vi "Panel.vi"(11 "DeviceArrayPanel in":refnum<class "DeviceArrayPanel.lvclass">) -> ()   [LabVIEW 2020, in "PicoG-App.lvlib" / "DeviceArrayPanel.lvclass"]
uses:
  DeviceArrayPanel.lvclass
  C:/Program Files (x86)/National Instruments/LabVIEW 2020/vi.lib/IlluminatedG/IG OOPanel/OOPanel/Panel/Panel.lvclass
  <vilib>/IlluminatedG/IG OOPanel/OOPanel/Panel/Basic UI State.ctl
  DeviceArrayPanel.lvclass/DeviceArrayPanel.ctl
  Device/Get ID.vi
  Device/Get Alias.vi
  Device/Get Platform Name.vi
  Device/Get Board.vi
  Device/Get Version String.vi
  <vilib>/IlluminatedG/IG OOPanel/OOPanel/Panel/Panel.lvclass
  <vilib>/IlluminatedG/IG OOPanel/OOPanel/OOPanel.lvlib
  Device/Device.lvclass
panel:
  out "ID":string="E6605838830B8539"
  out "Version String":string="0.0.3"
  out "Board":string="pico"
  out "Platform Name":string="RP2040"
  out "Alias":string="NomadPico"
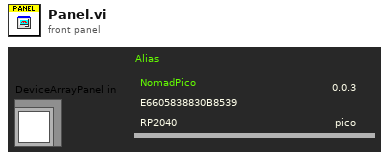
[diagram p1: front panel]
types:
  T1 = typedef "OOPanel.lvlib/Panel.lvclass/Basic UI State.ctl" = enum16{"Init", "Run", "Close"}
  T2 = typedef "PicoG-App.lvlib/DeviceArrayPanel.lvclass/Inbound Events.ctl" = cluster{"Device Set":refnum<user-event>, "Set Highlighted":refnum<user-event>}
  T3 = typedef "OOPanel.lvlib/Panel.lvclass/Panel Events.ctl" = cluster{"Visbility":refnum<user-event>, "Close":refnum<user-event>}
  T4 = typedef "PicoG-App.lvlib/DeviceArrayPanel.lvclass/Ref Data.ctl" = cluster{"Device":refnum<class "Device.lvclass">}
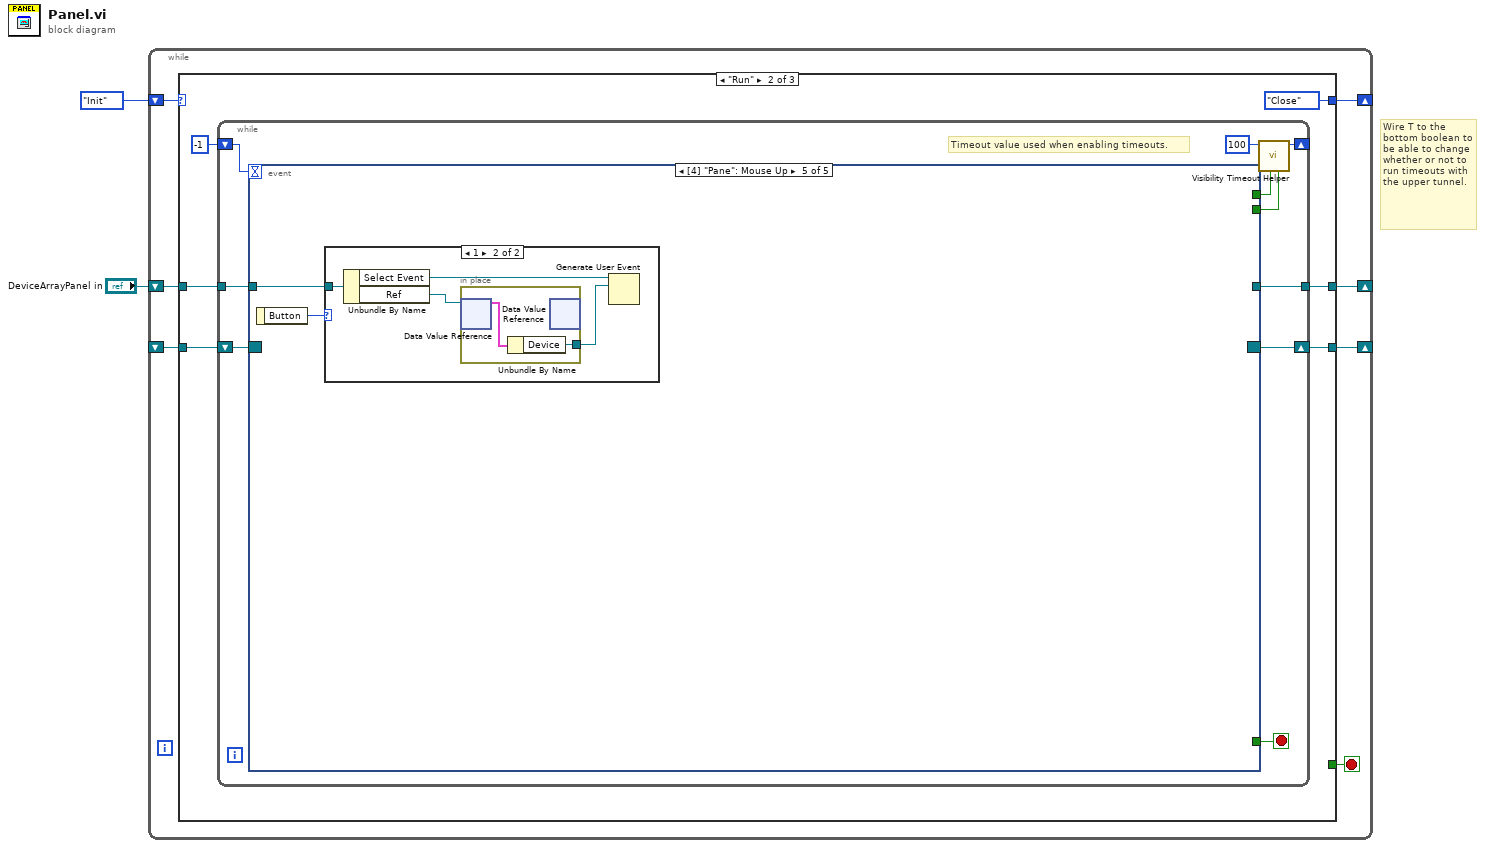
[diagram p0: block diagram]
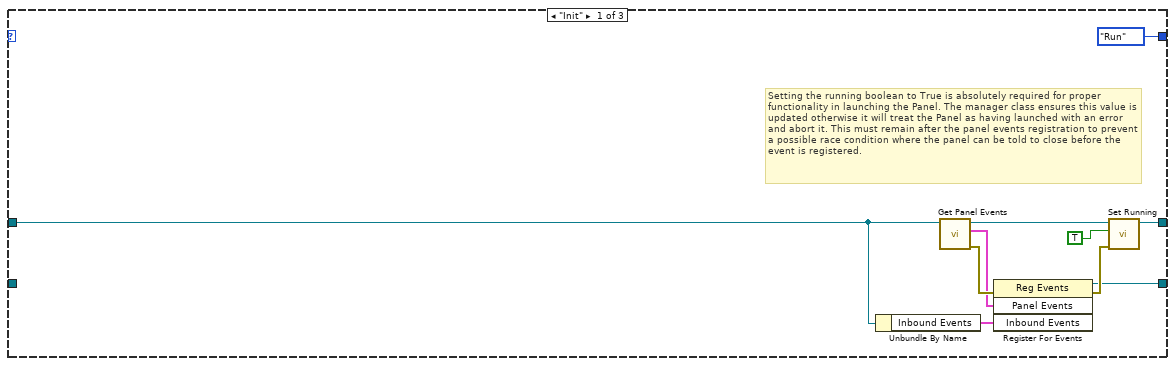
[diagram p2: hidden frame]
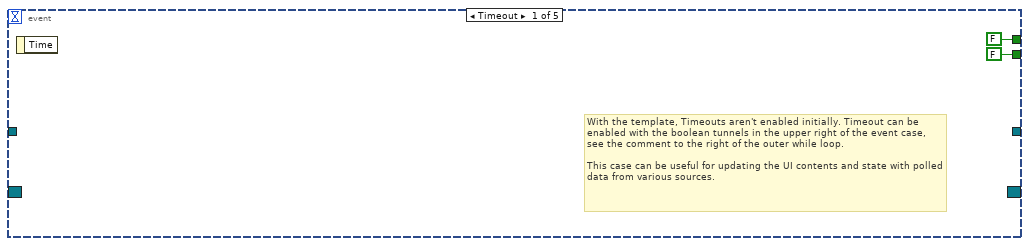
[diagram p3: hidden frame]
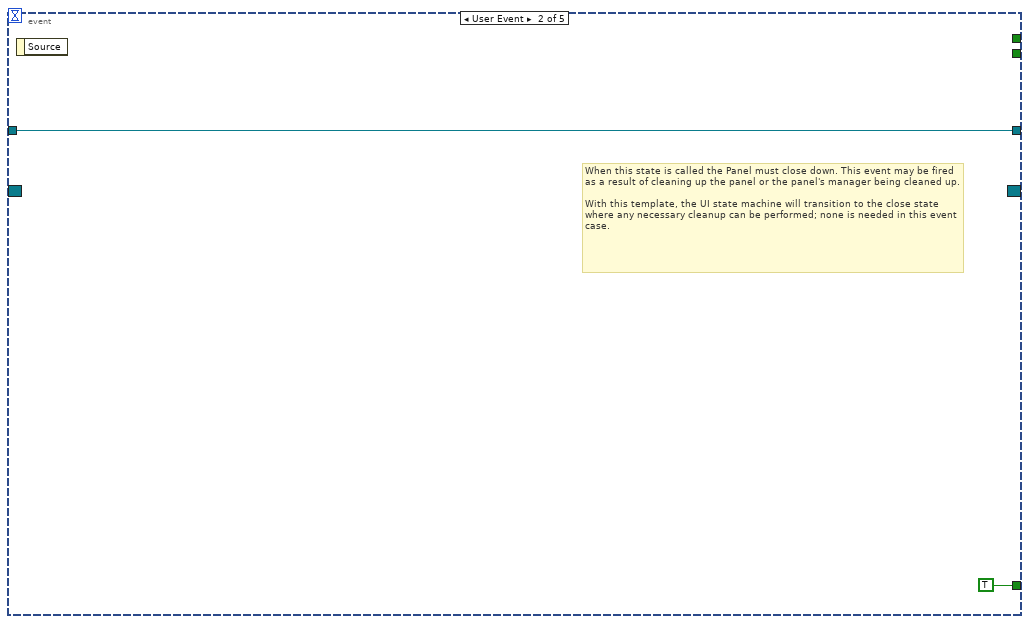
[diagram p4: hidden frame]
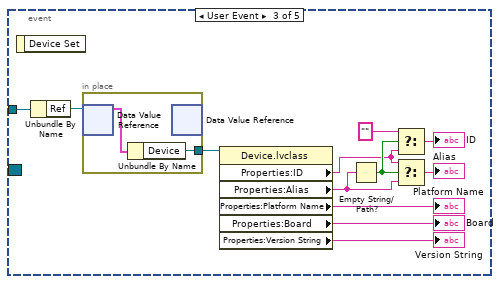
[diagram p5: hidden frame]
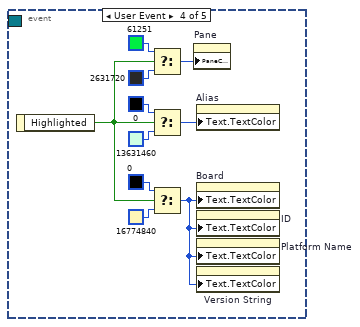
[diagram p6: hidden frame]
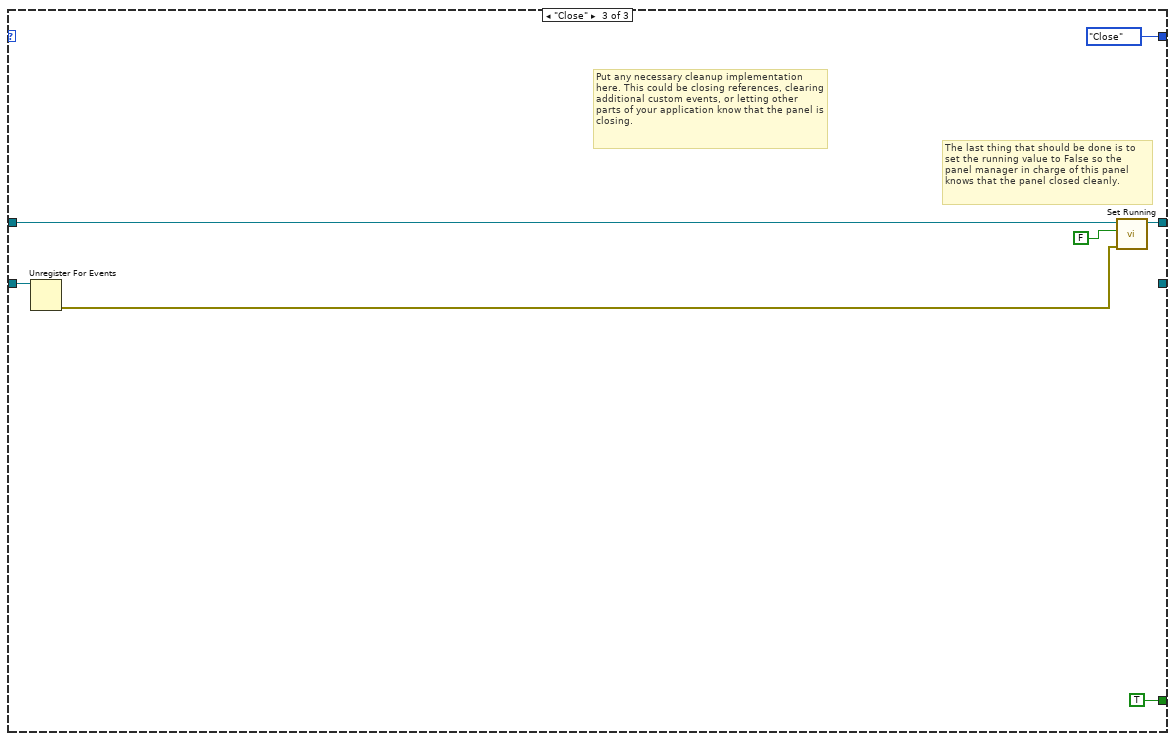
[diagram p8: hidden frame]
diagram:
  # "Wire T to the bottom boolean to be able to change whether or not to run timeouts with the upper tunnel."
  n1 = while {
    shift-right: [w8] -> _
    shift-left: _ -> [w9]
    shift-right: [w6] -> _
    shift-left: Basic_UI_State."Init" ("Basic UI State") -> [w7]
    shift-right: [w4] -> _
    shift-left: "DeviceArrayPanel in" -> [w3]
    stop <- w5 stop-if-true
    n2 = case shown="\"Run\"" w7 {
      tunnel: w9 -> [_ w25 w74]
      tunnel: [w13 w23 _] -> w8
      tunnel: [Basic_UI_State."Run" ("Basic UI State") Basic_UI_State."Close" ("Basic UI State") Basic_UI_State."Close" ("Basic UI State")] -> w6
      tunnel: [_ _ TRUE] -> w5
      tunnel: [w12 w20 w72] -> w4
      tunnel: w3 -> [w11 w21 w73]
      frame "Init" {
        # "Setting the running boolean to True is absolutely required for proper functionality in launching the Panel. The manager class ensures this value is updated otherwise it will treat the Panel as having launched with an error and abort it. This must remain after the panel events registration to prevent a possible race condition where the panel can be told to close before the event is registered."
        n3 = Unbundle By Name(w11) -> ("Inbound Events"=w10:T2)
        n4 = call <vilib>:"Get Panel Events.vi"("Panel in"=w11) -> ("error out"=w19:errorcluster, "Panel Events"=w15:T3, "Panel out"=w16:refnum<class "DeviceArrayPanel.lvclass">)  [unwired: 8 in]
        n5 = register-events(error in=w19, w15, w10) -> (reference out=w13:refnum<event-registration>, error out=w17:errorcluster)  [unwired: 1 in]
        n6 = call <vilib>:"Set Running.vi"("error in (no error)"=w17, "Running"=TRUE, "Panel in"=w16) -> ("Panel out"=w12:refnum<class "DeviceArrayPanel.lvclass">)  [unwired: 7 in, 1 out]
      }
      frame "Run" {
        n7 = while {
          shift-right: [w31] -> w23
          shift-left: w25 -> [w32]
          shift-right: [w34] -> _
          shift-left: -1 ("Timeout") -> [w33]
          tunnel: w21 -> [w27]
          tunnel: [w26] -> w20
          stop <- w28 stop-if-true
          # "Timeout value used when enabling timeouts."
          n8 = event shown="[4] \"Pane\": Mouse Up" {
            selector: w32 -> [_ _ _ _ _]
            dyn-events: [_ _ _ _ _] -> w31
            timeout: w33 -> [_ _ _ _ _]
            tunnel: [FALSE _ _ _ _] -> w30
            tunnel: [FALSE _ _ _ _] -> w29
            tunnel: [_ TRUE _ _ _] -> w28
            tunnel: w27 -> [_ w38 w50 _ w65]
            tunnel: [_ w38 _ _ _] -> w26
            event Timeout {
              # "With the template, Timeouts aren't enabled initially. Timeout can be enabled with the boolean tunnels in the upper right of the event case, see the comment to the right of the outer while loop.\n\nThis case can be useful for updating the UI contents and state with polled data from various sources."
              n9 = event-data() -> ()  [unwired: 1 in, 1 out]
            }
            event User Event {
              # "When this state is called the Panel must close down. This event may be fired as a result of cleaning up the panel or the panel's manager being cleaned up.\n\nWith this template, the UI state machine will transition to the close state where any necessary cleanup can be performed; none is needed in this event case."
              n10 = event-data() -> ()  [unwired: 1 in, 1 out]
            }
            event User Event {
              n11 = event-data() -> ()  [unwired: 1 in, 1 out]
              n12 = Unbundle By Name(w50) -> ("Ref"=w51:refnum<data-value>)
              n13 = in-place {
                in-place-border: [w52] -> w49
                n14 = in-place-dvr #1(w51) -> (w53:T4)  [unwired: 1 out]
                n15 = Unbundle By Name(w53) -> ("Device"=w52:refnum<class "Device.lvclass">)
                n16 = in-place-dvr #1() -> ()  [unwired: 1 in, 2 out]
              }
              n17 = property class="Device.lvclass"(reference=w49) -> ("Properties:ID"=w42:string, "Properties:Alias"=w48:string, "Properties:Platform Name"=→"Platform Name":string, "Properties:Board"=→"Board":string, "Properties:Version String"=→"Version String":string)  [unwired: 1 in, 2 out]
              n18 = Empty String/Path?(string/path=w48) -> (empty?=w43:bool)
              n19 = Select(t="", s=w43, f=w42) -> (s? t:f=→"ID":string)
              n20 = Select(t=w42, s=w43, f=w48) -> (s? t:f=→"Alias":string)
            }
            event User Event {
              n21 = event-data() -> ("Highlighted"=w55:bool)  [unwired: 1 in]
              n22 = Select(t=u32 61251, s=w55, f=u32 2631720) -> (s? t:f=w61:u32)
              n23 = Select(t=u32 0, s=w55, f=u32 13631460) -> (s? t:f=w58:u32)
              n24 = Select(t=u32 0, s=w55, f=u32 16774840) -> (s? t:f=w54:u32)
              n25 = property on="Pane" class="Pane"("PaneColor"=w61) -> ()  [unwired: 2 in, 2 out]
              n26 = property on="Alias" class="Str"("Text.TextColor"=w58) -> ()  [unwired: 2 in, 2 out]
              n27 = property on="Board" class="Str"("Text.TextColor"=w54) -> ()  [unwired: 2 in, 2 out]
              n28 = property on="ID" class="Str"("Text.TextColor"=w54) -> ()  [unwired: 2 in, 2 out]
              n29 = property on="Platform Name" class="Str"("Text.TextColor"=w54) -> ()  [unwired: 2 in, 2 out]
              n30 = property on="Version String" class="Str"("Text.TextColor"=w54) -> ()  [unwired: 2 in, 2 out]
            }
            event Mouse Up {
              n31 = event-data() -> ("Button"=w64:u16)  [unwired: 1 in]
              n32 = case shown="1" w64 {
                tunnel: w65 -> [_ w68]
                frame Default {
                }
                frame 1 {
                  n33 = Unbundle By Name(w68) -> ("Select Event"=w67:refnum<user-event>, "Ref"=w69:refnum<data-value>)
                  n34 = in-place {
                    in-place-border: [w70] -> w66
                    n35 = in-place-dvr #2(w69) -> (w71:T4)  [unwired: 1 out]
                    n36 = Unbundle By Name(w71) -> ("Device"=w70:refnum<class "Device.lvclass">)
                    n37 = in-place-dvr #2() -> ()  [unwired: 1 in, 2 out]
                  }
                  n38 = Generate User Event(user event=w67, event data cluster=w66) -> ()  [unwired: 2 in, 2 out]
                }
              }
            }
          }
          n39 = call <vilib>:"Visibility Timeout Helper.vi"("Update?"=w29, "Use Timeout?"=w30, "Visible Timeout mS"=100) -> ("Timeout"=w34:i32)  [unwired: 8 in]
        }
      }
      frame "Close" {
        # "Put any necessary cleanup implementation here. This could be closing references, clearing additional custom events, or letting other parts of your application know that the panel is closing."
        # "The last thing that should be done is to set the running value to False so the panel manager in charge of this panel knows that the panel closed cleanly."
        n40 = Unregister For Events(event registration refnum=w74) -> (error out=w76:errorcluster)  [unwired: 1 in]
        n41 = call <vilib>:"Set Running.vi"("error in (no error)"=w76, "Running"=FALSE, "Panel in"=w73) -> ("Panel out"=w72:refnum<class "DeviceArrayPanel.lvclass">)  [unwired: 7 in, 1 out]
      }
    }
  }
